vi "Add Calculate Channel_Lowpass Filter_Lowpass Filter.vi"(7 "SysDef Ref":T1, 8 "error in (error out)":errorcluster, 9 "Lowpass Filter Settings":T2={"Name"="", "Description"="", "Channel to Filter Node Path"="", "LowCutoffFrequency"=0.125, "FilterOrder"=1}, 11 "Calculated Channels Ref":refnum<k24>) -> (0 "error out":errorcluster, 3 "Calculated Channels Ref Out":refnum<k24>)   [LabVIEW 2019, in "Simple SysDef API.lvlib"]
uses:
  <userlib>/SimpleSysDef/Simple SysDef API.lvlib
  NationalInstruments.VeriStand.SystemDefinitionAPI
  <userlib>/SimpleSysDef/_SubVIs/Add Calculate Channel_Lowpass Filter_Settings.ctl
  <userlib>/SimpleSysDef/_SubVIs/System Definition Reference.ctl
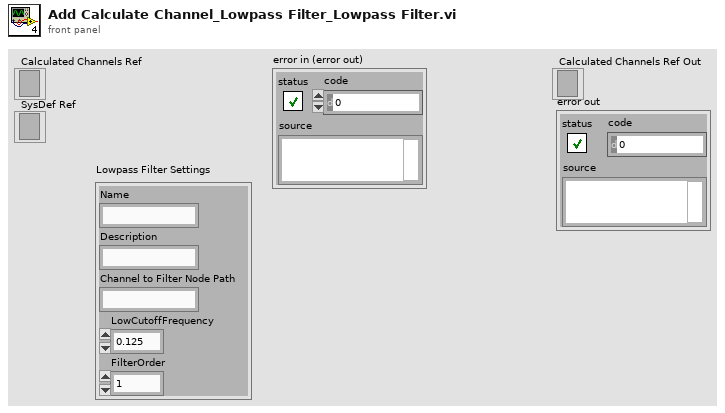
[diagram p1: front panel]
types:
  T1 = typedef "Simple SysDef API.lvlib/System Definition Reference.ctl" = refnum<k24>
  T2 = typedef "Simple SysDef API.lvlib/Add Calculate Channel_Lowpass Filter_Settings.ctl" = cluster{"Name":string, "Description":string, "Channel to Filter Node Path":string, "LowCutoffFrequency":dbl, "FilterOrder":i32}
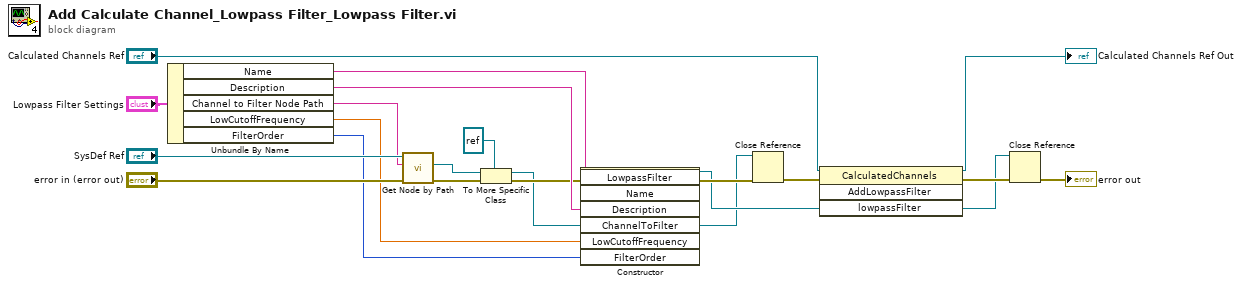
[diagram p0: block diagram]
diagram:
  n1 = Unbundle By Name("Lowpass Filter Settings") -> ("Name"=w10:string, "Description"=w9:string, "Channel to Filter Node Path"=w3:string, "LowCutoffFrequency"=w2:dbl, "FilterOrder"=w1:i32)
  n2 = call <userlib>:"Get Node by Path.vi"("error in (no error)"="error in (error out)", "System Definition Node Path"=w3, "SysDef Ref"="SysDef Ref") -> ("error out"=w6:errorcluster, "Node Ref"=w7:refnum<k24>)  [unwired: 6 in, 1 out]
  n3 = To More Specific Class(target class=refnum<k24> refnum ("ChannelToAverage"), reference=w7, error in=w6) -> (specific class reference=w4:refnum<k24>, error out=w5:errorcluster)
  n4 = constructor class="LowpassFilter"(error in=w5, "Name"=w10, "Description"=w9, "ChannelToFilter"=w4, "LowCutoffFrequency"=w2, "FilterOrder"=w1) -> (reference out=w11:refnum<k24>, error out=w13:errorcluster)  [unwired: 2 in, 6 out]
  n5 = Close Reference(reference=w4, error in (no error)=w13) -> (error out=w12:errorcluster)
  n6 = invoke class="CalculatedChannels" method="AddLowpassFilter"(reference="Calculated Channels Ref", error in=w12, "lowpassFilter"=w11) -> (reference out=→"Calculated Channels Ref Out":refnum<k24>, error out=w14:errorcluster)  [unwired: 1 in, 2 out]
  n7 = Close Reference(reference=w11, error in (no error)=w14) -> (error out=→"error out":errorcluster)
